vi "apply channel changes.vi"(8 "error in":errorcluster, 9 "new channel":refnum<class "TBM channel.lvclass">, 10 "old channel":refnum<class "TBM channel.lvclass">, 11 "UI Reference configuration in":refnum<class "io configuration.lvclass">) -> (0 "error out":errorcluster, 3 "UI Reference configuration out":refnum<class "io configuration.lvclass">)   [LabVIEW 2015, in "io configuration.lvclass"]
uses:
  io configuration.lvclass
  <vilib>/NI/Tag Bus Module Framework/channel/TBM channel.lvclass
  io configuration.lvclass/io configuration.ctl
  <vilib>/NI/Tag Bus/tag/tag descriptor.lvclass/tag descriptor.ctl
  <vilib>/NI/Tag Bus/tag/tag descriptor.lvclass
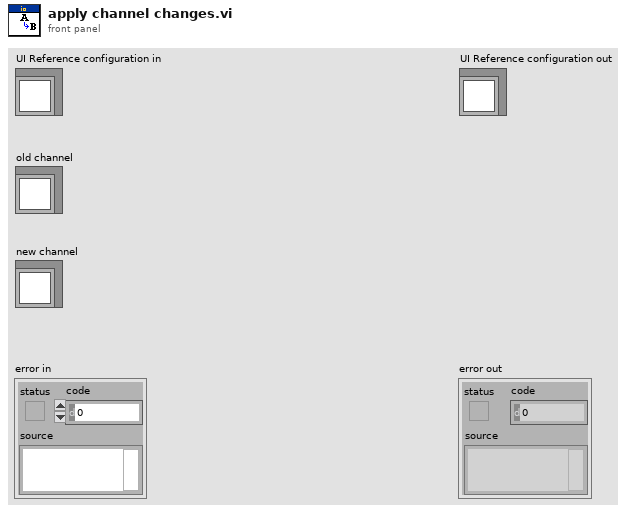
[diagram p1: front panel]
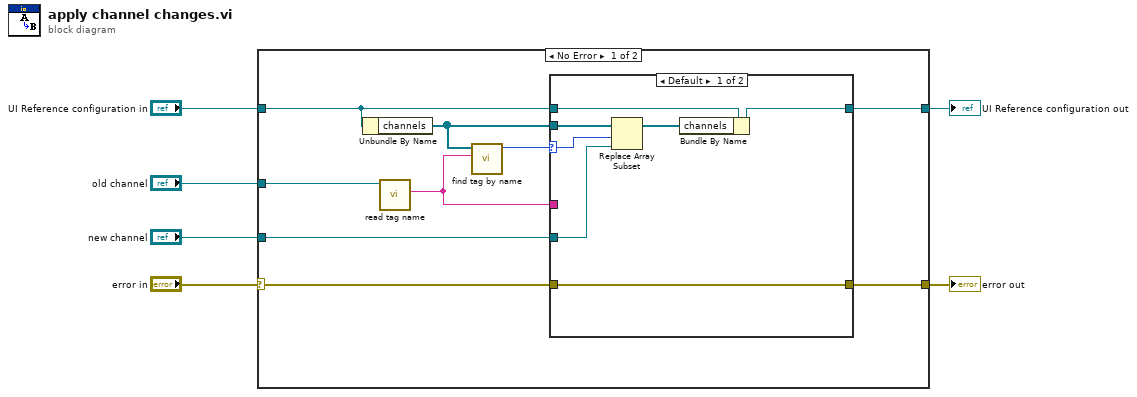
[diagram p0: block diagram]
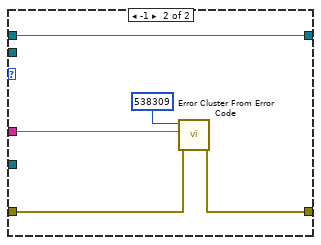
[diagram p2: hidden frame]
diagram:
  n1 = case shown="No Error" "error in" {
    selector: "error in" -> [w10 w29]
    tunnel: [w9 w29] -> w5
    tunnel: [w13 w28] -> w3
    tunnel: "UI Reference configuration in" -> [w14 w28]
    tunnel: "old channel" -> [w15 _]
    tunnel: "new channel" -> [w11 _]
    frame No Error {
      n2 = Unbundle By Name(w14) -> ("channels"=w12:refnum<class "TBM channel.lvclass">[])
      n3 = call <vilib>:"read tag name.vi"("system tag in"=w15) -> ("name"=w7:string)  [unwired: 8 in, 2 out]
      n4 = call <vilib>:"find tag by name.vi"("name"=w7, "tags in"=w12) -> ("index"=w8:i32)  [unwired: 9 in]
      n5 = case shown="Default" w8 {
        selector: w8 -> [w20 _]
        tunnel: w14 -> [w22 w27]
        tunnel: [w19 w27] -> w13
        tunnel: w12 -> [w21 _]
        tunnel: w11 -> [w17 _]
        tunnel: w7 -> [_ w25]
        tunnel: w10 -> [w16 w24]
        tunnel: [w16 w23] -> w9
        frame Default {
          n6 = Replace Array Subset(array=w21, new element=w17, index=w20) -> (w18:refnum<class "TBM channel.lvclass">[])
          n7 = Bundle By Name(cluster=w22, "channels"=w18) -> (w19:refnum<class "io configuration.lvclass">)
        }
        frame -1 {
          n8 = call <vilib>:"Error Cluster From Error Code.vi"("error in (no error)"=w24, "error message (\"\")"=w25, "error code (0)"=538309) -> ("error out"=w23:errorcluster)  [unwired: 6 in]
        }
      }
    }
    frame Error {
    }
  }
  "error out" <- w5
  "UI Reference configuration out" <- w3
